vi "HFRR ADV v011 new software.vi"() -> ()   [LabVIEW 2025] (continued)
            n341 = local write "Main Tab"(T2."About" ("Main Tab")) -> ()
            n342 = local write "Cal Password"("" ("Cal Password")) -> ()
            n343 = local write "Main Dashboard Buttons"(T1."About" ("Main Dashboard Buttons")) -> ()
            n344 = local write "Tab Control 5"(T11."Temperature Calibration" ("Tab Control 5")) -> ()
            n345 = property on="Calibration 2" class="TabCtl (strict)"("Visible"=FALSE) -> ()  [unwired: 2 in, 2 out]
            n346 = property on="Tab Control 5" class="TabCtl (strict)"("Tabs Visible?"=FALSE ("Page Labels Display Visible?")) -> ()  [unwired: 2 in, 2 out]
            n347 = local write "Calibration"(FALSE ("Calibration")) -> ()
          }
        }
      }
      event "Calibration Selection": Value Change {
        n348 = event-data() -> ()  [unwired: 1 in, 6 out]
        n349 = local read "Calibration Selection"() -> (w438:T8)
        n350 = case shown="Default" w438 {
          tunnel: [T7."Stroke" ("Main Calibration Tab") T7."Friction" ("Main Calibration Tab") T7."Main" ("Main Calibration Tab") T7."Temperature" ("Main Calibration Tab")] -> w437
          frame "Stroke Calibration" {
          }
          frame "Friction Force Calibration" {
          }
          frame Default {
          }
          frame "Temperature Calibration" {
          }
        }
        n351 = local write "Main Calibration Tab"(w437) -> ()
      }
      event "Back Stroke": Value Change {
        n352 = event-data() -> ()  [unwired: 1 in, 6 out]
        n353 = local write "Main Stroke Tab"(T9."Step 1" ("Main Stroke Tab")) -> ()
        n354 = local write "Main Calibration Tab"(T7."Main" ("Main Calibration Tab")) -> ()
        n355 = local write "Back Stroke"(FALSE ("Back Stroke")) -> ()
      }
      event "Step 2 Back": Value Change {
        n356 = event-data() -> ()  [unwired: 1 in, 6 out]
        n357 = local write "Main Stroke Tab"(T9."Step 1" ("Main Stroke Tab")) -> ()
        n358 = local write "Step 2 Back"(FALSE ("Back Stroke")) -> ()
      }
      event "Step 3 Back": Value Change {
        n359 = event-data() -> ()  [unwired: 1 in, 6 out]
        n360 = local write "Main Stroke Tab"(T9."Step 2" ("Main Stroke Tab")) -> ()
        n361 = local write "Step 3 Back"(FALSE ("Back Stroke")) -> ()
      }
      event "Step 4 Back": Value Change {
        n362 = event-data() -> ()  [unwired: 1 in, 6 out]
        n363 = local write "Main Stroke Tab"(T9."Step 3" ("Main Stroke Tab")) -> ()
        n364 = local write "Step 4 Back"(FALSE ("Back Stroke")) -> ()
      }
      event "Step 5 Back": Value Change {
        n365 = event-data() -> ()  [unwired: 1 in, 6 out]
        n366 = local write "Main Stroke Tab"(T9."Step 4" ("Main Stroke Tab")) -> ()
        n367 = local write "Step 5 Back"(FALSE ("Back Stroke")) -> ()
      }
      event "Step 6 Back": Value Change {
        n368 = event-data() -> ()  [unwired: 1 in, 6 out]
        n369 = local write "Main Stroke Tab"(T9."Step 5" ("Main Stroke Tab")) -> ()
        n370 = local write "Step 6 Back"(FALSE ("Back Stroke")) -> ()
      }
      event "Back Stroke step 7": Value Change {
        n371 = event-data() -> ()  [unwired: 1 in, 6 out]
        n372 = local write "Main Stroke Tab"(T9."Step 6" ("Main Stroke Tab")) -> ()
        n373 = local write "Back Stroke step 7"(FALSE ("Back Stroke")) -> ()
      }
      event "Back Stroke step 8": Value Change {
        n374 = event-data() -> ()  [unwired: 1 in, 6 out]
        n375 = local write "Main Stroke Tab"(T9."Step 7" ("Main Stroke Tab")) -> ()
        n376 = local write "Back Stroke step 8"(FALSE ("Back Stroke")) -> ()
      }
      event "Back Stroke 8": Value Change {
        n377 = event-data() -> ()  [unwired: 1 in, 6 out]
        n378 = local write "Main Stroke Tab"(T9."Step 1" ("Main Stroke Tab")) -> ()
        n379 = local write "Back Stroke 8"(FALSE ("Back Stroke 8")) -> ()
      }
      event "Continue Stroke": Value Change {
        n380 = event-data() -> ()  [unwired: 1 in, 6 out]
        n381 = local write "Main Stroke Tab"(T9."Step 2" ("Main Stroke Tab")) -> ()
        n382 = local write "Continue Stroke"(FALSE ("Continue Stroke")) -> ()
      }
      event "Continue Stroke step 2": Value Change {
        n383 = event-data() -> ()  [unwired: 1 in, 6 out]
        n384 = local write "Main Stroke Tab"(T9."Step 3" ("Main Stroke Tab")) -> ()
        n385 = local write "Continue Stroke step 2"(FALSE ("Continue Stroke")) -> ()
      }
      event "Continue Stroke step 3": Value Change {
        n386 = event-data() -> ()  [unwired: 1 in, 6 out]
        n387 = local write "Main Stroke Tab"(T9."Step 4" ("Main Stroke Tab")) -> ()
        n388 = local write "Continue Stroke step 3"(FALSE ("Continue Stroke")) -> ()
      }
      event "Continue Stroke step 4": Value Change {
        n389 = event-data() -> ()  [unwired: 1 in, 6 out]
        n390 = local write "Main Stroke Tab"(T9."Step 5" ("Main Stroke Tab")) -> ()
        n391 = local write "Continue Stroke step 4"(FALSE ("Continue Stroke")) -> ()
      }
      event "Continue Stroke step 5": Value Change {
        n392 = event-data() -> ()  [unwired: 1 in, 6 out]
        n393 = local write "Main Stroke Tab"(T9."Step 6" ("Main Stroke Tab")) -> ()
        n394 = local write "Continue Stroke step 5"(FALSE ("Continue Stroke")) -> ()
      }
      event "Continue Stroke step 6": Value Change {
        n395 = event-data() -> ()  [unwired: 1 in, 6 out]
        n396 = local write "Main Stroke Tab"(T9."Step 7" ("Main Stroke Tab")) -> ()
        n397 = local write "Continue Stroke step 6"(FALSE ("Continue Stroke")) -> ()
      }
      event "Continue Stroke step 7": Value Change {
        w475 = FALSE ("0.2mm")
        n398 = event-data() -> ()  [unwired: 1 in, 6 out]
        n399 = local write "0.4 mm"(w475) -> ()
        n400 = local write "0.6 mm"(w475) -> ()
        n401 = local write "1.0 mm"(w475) -> ()
        n402 = local write "1.2 mm"(w475) -> ()
        n403 = local write "0.2 2"(w475) -> ()
        n404 = local write "0.4 2"(w475) -> ()
        n405 = local write "0.6 2"(w475) -> ()
        n406 = local write "0.8 2"(w475) -> ()
        n407 = local write "1.0 2"(w475) -> ()
        n408 = local write "1.2"(w475) -> ()
        n409 = local write "0.2mm"(w475) -> ()
        n410 = local write "0.8mm"(w475) -> ()
        n411 = local write "Main Stroke Tab"(T9."Step 8" ("Main Stroke Tab")) -> ()
        n412 = local write "Continue Stroke step 7"(FALSE ("Continue Stroke")) -> ()
        n413 = local write "Stroke Test Complete"(T10."Test Progress" ("Stroke Test Complete")) -> ()
        "Position Measurment Temp" <- 0.0 ("Position Measurment Temp")
        "Calibration Tare" <- TRUE ("Calibration Tare")
      }
      event "Continue Stroke step 8": Value Change {
        n414 = event-data() -> ()  [unwired: 1 in, 6 out]
        n415 = local read "LVDT STROKE  Calibration"() -> (w480:dbl)
        n416 = local read "Position Measurment Temp"() -> (w481:dbl)
        n417 = case shown="0, Default" w481 {
          selector: w481 -> [w486 w491 w496 w501 w506 w511 w514 w517]
          tunnel: w480 -> [w482 w487 w492 w497 w502 w507 _ _]
          frame 0, Default {
            w484 = TRUE ("0.2mm")
            n418 = Increment(x=w486) -> (x+1=w485:i32)
            n419 = local write "Position Measurment Temp"(w485) -> ()
            n420 = local write "0.2mm"(w484) -> ()
            n421 = local write "0.2 2"(w484) -> ()
            n422 = local write "MOVE CARRIAGE TO"(0.2 ("MOVE CARRIAGE TO")) -> ()
            "Calibration 0.2" <- w482
          }
          frame 1 {
            w489 = TRUE ("0.4 mm")
            n423 = Increment(x=w491) -> (x+1=w490:i32)
            n424 = local write "Calibration 0.4"(w487) -> ()
            n425 = local write "Position Measurment Temp"(w490) -> ()
            n426 = local write "0.4 mm"(w489) -> ()
            n427 = local write "MOVE CARRIAGE TO"(0.4 ("MOVE CARRIAGE TO")) -> ()
            n428 = local write "0.4 2"(w489) -> ()
          }
          frame 2 {
            w494 = TRUE ("0.6 mm")
            n429 = Increment(x=w496) -> (x+1=w495:i32)
            n430 = local write "Calibration 0.6"(w492) -> ()
            n431 = local write "Position Measurment Temp"(w495) -> ()
            n432 = local write "0.6 2"(w494) -> ()
            n433 = local write "0.6 mm"(w494) -> ()
            n434 = local write "MOVE CARRIAGE TO"(0.6 ("MOVE CARRIAGE TO")) -> ()
          }
          frame 3 {
            w498 = TRUE ("0.6 mm")
            n435 = Increment(x=w501) -> (x+1=w500:i32)
            n436 = local write "Position Measurment Temp"(w500) -> ()
            n437 = local write "MOVE CARRIAGE TO"(0.8 ("MOVE CARRIAGE TO")) -> ()
            n438 = local write "0.8mm"(w498) -> ()
            n439 = local write "0.8 2"(w498) -> ()
            "Calibration 0.8" <- w497
          }
          frame 4 {
            w503 = TRUE ("0.6 mm")
            n440 = Increment(x=w506) -> (x+1=w505:i32)
            n441 = local write "Position Measurment Temp"(w505) -> ()
            n442 = local write "MOVE CARRIAGE TO"(1.0 ("MOVE CARRIAGE TO")) -> ()
            n443 = local write "1.0 mm"(w503) -> ()
            n444 = local write "1.0 2"(w503) -> ()
            "Calibration 1.0" <- w502
          }
          frame 5 {
            w508 = TRUE ("0.6 mm")
            n445 = Increment(x=w511) -> (x+1=w510:i32)
            n446 = local write "Position Measurment Temp"(w510) -> ()
            n447 = local write "MOVE CARRIAGE TO"(1.2 ("MOVE CARRIAGE TO")) -> ()
            n448 = local write "1.2 mm"(w508) -> ()
            n449 = local write "1.2"(w508) -> ()
            "Calibration 1.2" <- w507
          }
          frame 6 {
            n450 = Increment(x=w514) -> (x+1=w513:i32)
            n451 = local write "Position Measurment Temp"(w513) -> ()
            n452 = local write "Stroke Test Complete"(T10."Stroke Points Completed" ("Stroke Test Complete")) -> ()
          }
          frame 7 {
            n453 = Increment(x=w517) -> (x+1=w516:i32)
            n454 = local write "Position Measurment Temp"(w516) -> ()
            n455 = local write "Main Stroke Tab"(T9."Step 9" ("Main Stroke Tab")) -> ()
          }
        }
      }
      event "Quit": Value Change {
        n456 = event-data() -> ()  [unwired: 1 in, 6 out]
      }
    }
    n457 = Wait (ms)(milliseconds to wait=u32 100) -> ()  [unwired: 1 out]
  }
  n458 = local write "Auto stop temp"(w14) -> ()
  n459 = while {
    stop <- w520 stop-if-true
    n460 = Wait (ms)(milliseconds to wait=u32 200) -> ()  [unwired: 1 out]
    n461 = local read "Quit"() -> (w520:bool)
  }
  n462 = local write "main tab sub"(enum32{"Page 1", "Page 2"}."Page 1" ("main tab sub")) -> ()
  n463 = local write "USERNAME"(w31) -> ()
  n464 = local write "Main Tab"(T2."HOME" ("Main Tab")) -> ()
  n465 = local write "USER ID"(w31) -> ()
  n466 = property on="Auto Scar Check  2" class="Clust (strict)"("Visible"=w14) -> (error out=w17:errorcluster)  [unwired: 2 in, 1 out]
  n467 = property on="Quit" class="Bool (strict)"("Value"=FALSE ("Quit")) -> (error out=w33:errorcluster)  [unwired: 2 in, 1 out]
  n468 = while {
    shift-right: [w522] -> _
    shift-left: "Enum - Selector" -> [w523]
    stop <- w524 stop-if-true
    # "Auto Start Logic Loop"
    n469 = case shown="\"close\"" w523 {
      tunnel: [w527 w533 w560 w592 w622 Auto_Start_enum."Exit" ("Enum - Selector") Auto_Start_enum."Init" ("Enum - Selector")] -> w522
      frame "Init", Default {
        n470 = local read "Auto Start Test"() -> (w526:bool)
        n471 = Select(t=Auto_Start_enum."Humidity & Temperature On" ("Enum - Selector"), s=w526, f=Auto_Start_enum."Init") -> (s? t:f=w527:T14)
      }
      frame "Humidity & Temperature On" {
        n472 = stacked-sequence {
          tunnel: [_ _ _ _ _ _ Auto_Start_enum."Reach point" ("Enum - Selector")] -> w530
          frame #0 {
            w535 = T17."Disabled and Grayed Out" ("Disabled")
            w536 = TRUE ("Heater Button")
            n473 = property on="Humidity" class="Bool (strict)"("DisabledEnum"=w535) -> ()  [unwired: 2 in, 2 out]
            n474 = property on="Heater Button" class="Bool (strict)"("DisabledEnum"=w535) -> ()  [unwired: 2 in, 2 out]
            n475 = local write "Heater Button"(w536) -> ()
            n476 = local write "Humidity"(w536) -> ()
            n477 = property on="Heater Button" class="Bool (strict)"("Val(Sgnl)"=TRUE ("Value (Signaling)")) -> ()  [unwired: 2 in, 2 out]
          }
          frame #1 {
            n478 = Wait (ms)(milliseconds to wait=u32 3000) -> ()  [unwired: 1 out]
          }
          frame #2 {
            n479 = local read "Set Temp"() -> (w542:dbl)
            n480 = Number To Fractional String(number=w542, precision (6)=i16 2) -> (F-format string=w539:string)  [unwired: 2 in]
            n481 = Concatenate Strings("ST;" ("Command"), w539) -> (w540:string)
            n482 = local write "Command"(w540) -> ()
          }
          frame #3 {
            n483 = Wait (ms)(milliseconds to wait=u32 1500) -> ()  [unwired: 1 out]
          }
          frame #4 {
            (unwired) i16 2 ("precision (6)")
            n484 = local read "Set Rh"() -> (w545:dbl)
            n485 = Number To Fractional String(number=w545) -> (F-format string=w548:string)  [unwired: 3 in]
            n486 = local read "WriteHumidity"() -> (w546:string[])
            n487 = Concatenate Strings("M;" ("new element/subarray"), w548) -> (w549:string)
            n488 = local write "Command"("HE;1" ("Command")) -> ()
            n489 = Insert Into Array(array=w546, new element=w549) -> (w547:string[])  [unwired: 1 in]
            n490 = local write "WriteHumidity"(w547) -> ()
          }
          frame #5 {
            n491 = Wait (ms)(milliseconds to wait=u32 1500) -> ()  [unwired: 1 out]
          }
          frame #6 {
            w552 = TRUE ("Reach point temp")
            n492 = local write "Reach point Humidity"(w552) -> ()
            n493 = local write "Reach point temp"(w552) -> ()
          }
        }
        n494 = local read "Auto Start Test"() -> (w532:bool)
        n495 = Not(x=w532) -> (.not. x?=w531:bool)
        n496 = Select(t=Auto_Start_enum."close", s=w531, f=w530) -> (s? t:f=w533:T14)
      }
      frame "Reach point" {
        w561 = TRUE ("PAUSE")
        w569 = 1.0 ("y")
        w572 = 1.0 ("y")
        n497 = local read "Set Temp"() -> (w554:dbl)
        n498 = local read "Set Humidity:"() -> (w568:dbl)
        n499 = local read "Humidity ( %RH )"() -> (w573:dbl)
        n500 = Add(x=w554, y=w572) -> (x+y=w571:dbl)
        n501 = Subtract(x=w554, y=w572) -> (x-y=w570:dbl)
        n502 = Add(x=w568, y=w569) -> (x+y=w567:dbl)
        n503 = Subtract(x=w568, y=w569) -> (x-y=w566:dbl)
        n504 = local read "TEMP"() -> (w574:dbl)
        n505 = In Range and Coerce(upper limit=w567, x=w573, lower limit=w566) -> (In Range?=w555:bool)  [unwired: 1 out]
        n506 = In Range and Coerce(upper limit=w571, x=w574, lower limit=w570) -> (In Range?=w556:bool)  [unwired: 1 out]
        n507 = case shown="True" w555 {
          frame False {
          }
          frame True {
            n508 = case shown="True" "Reach point Humidity" {
              selector: "Reach point Humidity" -> [_ w580]
              frame False {
              }
              frame True {
                n509 = local read "EVENT LOG"() -> (w577:string)
                n510 = Not(x=w580) -> (.not. x?=w579:bool)
                n511 = local write "Reach point Humidity"(w579) -> ()
                n512 = call "Event Log.vi"("Content"="Target Humidity reached", "EVENT LOG"=w577) -> ("EVENT LOG"=w578:string)  [unwired: 8 in, 1 out]
                n513 = local write "EVENT LOG"(w578) -> ()
              }
            }
          }
        }
        n514 = case shown="True" w556 {
          frame False {
          }
          frame True {
            n515 = case shown="True" "Reach point temp" {
              selector: "Reach point temp" -> [_ w586]
              frame False {
              }
              frame True {
                n516 = local read "EVENT LOG"() -> (w583:string)
                n517 = Not(x=w586) -> (.not. x?=w585:bool)
                n518 = local write "Reach point temp"(w585) -> ()
                n519 = call "Event Log.vi"("Content"="Target Temperature reached", "EVENT LOG"=w583) -> ("EVENT LOG"=w584:string)  [unwired: 8 in, 1 out]
                n520 = local write "EVENT LOG"(w584) -> ()
              }
            }
          }
        }
        n521 = local read "Auto Start Test"() -> (w559:bool)
        n522 = And(x=w556, y=w555) -> (x .and. y?=w565:bool)
        n523 = Select(t=Auto_Start_enum."Maintain Stage" ("Enum - Selector"), s=w565, f=Auto_Start_enum."Reach point" ("Enum - Selector")) -> (s? t:f=w562:T14)
        n524 = Not(x=w559) -> (.not. x?=w558:bool)
        n525 = Select(t=Auto_Start_enum."close", s=w558, f=w562) -> (s? t:f=w560:T14)
        n526 = call "ELAPSED TIMER VI.vi"("RESET"=w561, "PAUSE"=w561) -> ()  [unwired: 7 in, 3 out]
      }
      frame "Maintain Stage" {
        w601 = 2.0 ("y")
        w600 = 1.0 ("y")
        # "Humidity and  temperatures Set Point  have been reached"
        n527 = local read "Set Temp"() -> (w587:dbl)
        n528 = local read "Set Humidity:"() -> (w604:dbl)
        n529 = local read "Humidity ( %RH )"() -> (w607:dbl)
        n530 = Add(x=w587, y=w600) -> (x+y=w606:dbl)
        n531 = Subtract(x=w587, y=w600) -> (x-y=w605:dbl)
        n532 = local read "TEMP"() -> (w608:dbl)
        n533 = Add(x=w604, y=w601) -> (x+y=w603:dbl)
        n534 = Subtract(x=w604, y=w601) -> (x-y=w602:dbl)
        n535 = In Range and Coerce(upper limit=w606, x=w608, lower limit=w605) -> (In Range?=w599:bool)  [unwired: 1 out]
        n536 = In Range and Coerce(upper limit=w603, x=w607, lower limit=w602) -> (In Range?=w598:bool)  [unwired: 1 out]
        n537 = And(x=w599, y=w598) -> (x .and. y?=w597:bool)
        n538 = Not(x=w597) -> (.not. x?=w596:bool)
        n539 = call "ELAPSED TIMER VI.vi"("TARGET"=60.0, "RESET"=w596, "PAUSE"=FALSE) -> ("ELAPSED INDICATION"=w593:bool)  [unwired: 6 in, 2 out]
        n540 = case shown="True" w593 {
          tunnel: w593 -> [_ w611]
          tunnel: [Auto_Start_enum."Maintain Stage" ("Enum - Selector") w610] -> w591
          frame False {
          }
          frame True {
            n541 = stacked-sequence {
              tunnel: w611 -> [_ _ _ _ _]
              tunnel: [_ _ _ _ Auto_Start_enum."Start Stage" ("Enum - Selector")] -> w610
              frame #0 {
                n542 = local read "EVENT LOG"() -> (w613:string)
                n543 = call "Event Log.vi"("Content"="Humidity and temperature set point has stabilized.", "EVENT LOG"=w613) -> ("EVENT LOG"=w614:string)  [unwired: 8 in, 1 out]
                n544 = local write "EVENT LOG"(w614) -> ()
              }
              frame #1 {
                n545 = Wait (ms)(milliseconds to wait=u32 100) -> ()  [unwired: 1 out]
              }
              frame #2 {
                n546 = local read "EVENT LOG"() -> (w617:string)
                n547 = call "Event Log.vi"("Content"="Auto Test Started", "EVENT LOG"=w617) -> ("EVENT LOG"=w618:string)  [unwired: 8 in, 1 out]
                n548 = local write "EVENT LOG"(w618) -> ()
              }
              frame #3 {
                w619 = TRUE ("RUN")
                n549 = local write "RUN"(w619) -> ()
                n550 = property on="Auto Start Temp" class="Bool (strict)"("Val(Sgnl)"=w619) -> ()  [unwired: 2 in, 2 out]
                "Auto Start Temp" <- w619
              }
              frame #4 {
              }
            }
          }
        }
        n551 = local read "Auto Start Test"() -> (w590:bool)
        n552 = Not(x=w590) -> (.not. x?=w589:bool)
        n553 = Select(t=Auto_Start_enum."close", s=w589, f=w591) -> (s? t:f=w592:T14)
      }
      frame "Start Stage" {
        w621 = TRUE ("PAUSE")
        n554 = local read "Auto Start Test"() -> (w626:bool)
        n555 = Not(x=w626) -> (.not. x?=w625:bool)
        n556 = Select(t=Auto_Start_enum."close" ("Enum - Selector"), s=w625, f=Auto_Start_enum."Start Stage" ("Enum - Selector")) -> (s? t:f=w622:T14)
        n557 = call "ELAPSED TIMER VI.vi"("RESET"=w621, "PAUSE"=w621) -> ()  [unwired: 7 in, 3 out]
      }
      frame "close" {
        w628 = FALSE ("Heater Button")
        n558 = local write "RUN"(w628) -> ()
        n559 = local write "Heater Button"(w628) -> ()
        n560 = local write "Humidity"(w628) -> ()
        n561 = local write "Auto Start Test"(w628) -> ()
        n562 = property on="Heater Button" class="Bool (strict)"("Val(Sgnl)"=FALSE ("Value (Signaling)")) -> ()  [unwired: 2 in, 2 out]
      }
      frame "Exit" {
      }
    }
    n563 = Wait (ms)(milliseconds to wait=u32 100) -> ()  [unwired: 1 out]
    n564 = local read "Quit"() -> (w524:bool)
  }
  n565 = property on="Service Password Log" class="Str"("Visible"=w14) -> ()  [unwired: 2 in, 2 out]
  n566 = property on="Password 3" class="Clust (strict)"("Visible"=w14) -> ()  [unwired: 2 in, 2 out]
  n567 = while {
    stop <- w657 stop-if-true
    w640 = errorcluster {"status"=FALSE, "code"=0, "source"=""} ("error in (no error) 3")
    # "this loop is for manual report generation"
    n568 = local read "Confirm Measrurement"() -> (w639:bool)
    n569 = case shown="True" w639 {
      selector: w639 -> [_ w747]
      tunnel: errorcluster {"status"=FALSE, "code"=0, "source"=""} ("error in (no error) 3") -> [_ w748]
      tunnel: [_ w746] -> _
      frame False {
      }
      frame True {
        n570 = stacked-sequence {
          tunnel: w748 -> [_ w781 _]
          tunnel: w747 -> [_ _ w888]
          tunnel: [_ w769 _] -> w746
          frame #0 {
            n571 = String To Path(string="C:\\LAB-IQ\\Image Calibrate v01.dcf") -> (path=w751:path)
            n572 = Open/Create/Replace File ("Open File")(file path (use dialog)=w751) -> (refnum out=w752:refnum<file>)  [unwired: 5 in, 2 out]
            n573 = for {
              N: 4 -> [_]
              tunnel: w752 -> [w758]
              i -> [w754]
              n574 = Read from Text File ("Read File")(file (use dialog)=w758) -> (text=w759:string)  [unwired: 3 in, 3 out]
              n575 = String Subset(string=w759, offset (0)=6, length (rest)=10 ("length (rest)")) -> (substring=w755:string)
              n576 = Fract/Exp String To Number(string=w755) -> (number=w753:dbl)  [unwired: 3 in, 1 out]
              n577 = case shown="3" w754 {
                tunnel: w753 -> [w760 w761 _ w762 _]
                frame 0 {
                  n578 = local write "5x Gain"(w760) -> ()
                }
                frame 1 {
                  n579 = local write "10x Gain"(w761) -> ()
                }
                frame 2 {
                }
                frame 3 {
                  n580 = local write "100x gain"(w762) -> ()
                }
                frame 4, Default {
                }
              }
            }
          }
          frame #1 {
            n581 = local read "TEST STANDARD"() -> (w764:T3)
            n582 = case shown="\"ISO 12156\"" w764 {
              tunnel: ["ASTM D6079" "ISO 12156"] -> w763
              frame "ASTM D6079", Default {
              }
              frame "ISO 12156" {
              }
            }
            n583 = call "IMAGE ANALYSIS.vi"("Enum"=POST_ANALYSIS_ENUM."GET MEASUREMENTS", "error in"=w781) -> ("error out"=w788:errorcluster)  [unwired: 8 in, 1 out]
            n584 = local read "Magnification :"() -> (w774:string)
            n585 = call "Stall Data Flow.vim"("value in"=w788, "milliseconds to wait"=u32 1000) -> ("value out"=w787:errorcluster)  [unwired: 1 out]
            n586 = local read "Test File List :"() -> (w785:string)
            n587 = case shown="\"10x\"" w774 {
              tunnel: [w824 w825] -> w772
              frame "5x", Default {
                n588 = local read "5x Gain"() -> (w824:dbl)
              }
              frame "10x" {
                # "5x"
                n589 = local read "10x Gain"() -> (w825:dbl)
              }
            }
            n590 = call "IMAGE ANALYSIS.vi"("Enum"=POST_ANALYSIS_ENUM."READ", "error in"=w787) -> ("error out"=w784:errorcluster, "data out"=w775:string)  [unwired: 8 in]
            n591 = Match Pattern(string=w775, regular expression="\"type\": ") -> (after substring=w779:string)  [unwired: 1 in, 3 out]
            n592 = call "IMAGE PATH CREATION PY.vi"("error in (no error)"=w784, "File Name :"=w785) -> ("error out"=w783:errorcluster, "File Path"=w771:path, "File Path String:"=w766:string)  [unwired: 7 in]
            n593 = Match Pattern(string=w779, regular expression=",") -> (before substring=w765:string)  [unwired: 1 in, 3 out]
            n594 = local read "Calibration Tab"() -> (w768:enum32{"Measrument", "Calibrate"})
            n595 = call "Stall Data Flow.vim"("value in"=w783, "milliseconds to wait"=u32 250) -> ("value out"=w767:errorcluster)  [unwired: 1 out]
            n596 = Equal?(x=w765, y="\"rectangle\"") -> (x = y?=w776:bool)
            n597 = case shown="False" w776 {
              tunnel: w775 -> [w830 w885]
              tunnel: w772 -> [_ w876]
              tunnel: cluster{"major":dbl, "minor":dbl, "average":dbl} {"major"=0.0, "minor"=0.0, "average"=0.0} -> [w828 w872]
              tunnel: [w827 w869] -> w770
              tunnel: w765 -> [w829 _]
              tunnel: w772 -> [w826 _]
              frame False {
                n598 = Equal?(x=w829, y="\"line\"") -> (x = y?=w831:bool)
                n599 = case shown="True" w831 {
                  tunnel: w830 -> [_ w846]
                  tunnel: w828 -> [w833 w845]
                  tunnel: [w833 w843] -> w827
                  tunnel: w826 -> [_ w842]
                  frame False {
                  }
                  frame True {
                    w841 = 0.0 ("Major Axis")
                    n600 = Match Pattern(string=w846, regular expression="\"length_px\":") -> (after substring=w844:string)  [unwired: 1 in, 3 out]
                    n601 = property on="Major Axis" class="DigNum (strict)"("Caption.Text"="") -> ()  [unwired: 2 in, 2 out]
                    n602 = property on="Minor Axis" class="DigNum (strict)"("Caption.Text"="") -> ()  [unwired: 2 in, 2 out]
                    n603 = property on="Average" class="DigNum (strict)"("Caption.Text"="Line") -> ()  [unwired: 2 in, 2 out]
                    n604 = Fract/Exp String To Number(string=w844, default (0 dbl)=0.0 ("default (0 DBL)")) -> (number=w840:dbl)  [unwired: 2 in, 1 out]
                    "Pixel Value" <- w840
                    n605 = Multiply(x=w840, y=w842) -> (x*y=w853:dbl)
                    n606 = Multiply(x=w853, y=1000.0) -> (x*y=w836:dbl)
                    n607 = Divide(x=w836, y=1000.0) -> (x/y=w839:dbl)
                    n608 = local write "Measurment (mm)"(w839) -> ()
                    n609 = Bundle By Name(cluster=w845, "average"=w836) -> (w843:cluster{"major":dbl, "minor":dbl, "average":dbl})
                    n610 = Number To Fractional String(number=w836, precision (6)=i16 1) -> (F-format string=w835:string)  [unwired: 2 in]
                    n611 = local write "Minor Axis"(w841) -> ()
                    n612 = local write "Major Axis"(w841) -> ()
                    n613 = Fract/Exp String To Number(string=w835) -> (number=w834:dbl)  [unwired: 3 in, 1 out]
                    n614 = local write "Average"(w834) -> ()
                  }
                }
              }
              frame True {
                w873 = 1000.0 ("y")
                w879 = 0.0 ("default (0 DBL)")
                n615 = Match Pattern(string=w885, regular expression=" \"width_px\":") -> (after substring=w883:string)  [unwired: 1 in, 3 out]
                n616 = Match Pattern(string=w883, regular expression="\"height_px\":") -> (before substring=w881:string, after substring=w880:string)  [unwired: 1 in, 2 out]
                n617 = Fract/Exp String To Number(string=w881, default (0 dbl)=w879) -> (number=w878:dbl)  [unwired: 2 in, 1 out]
                n618 = Fract/Exp String To Number(string=w880, default (0 dbl)=w879) -> (number=w877:dbl)  [unwired: 2 in, 1 out]
                n619 = Multiply(x=w878, y=w876) -> (x*y=w875:dbl)
                n620 = Multiply(x=w877, y=w876) -> (x*y=w874:dbl)
                n621 = Multiply(x=w875, y=w873) -> (x*y=w859:dbl)
                n622 = Multiply(x=w874, y=w873) -> (x*y=w857:dbl)
                n623 = Add(x=w859, y=w857) -> (x+y=w871:dbl)
                n624 = property on="Major Axis" class="DigNum (strict)"("Caption.Text"="Major Axis") -> ()  [unwired: 2 in, 2 out]
                n625 = property on="Minor Axis" class="DigNum (strict)"("Caption.Text"="Minor Axis") -> ()  [unwired: 2 in, 2 out]
                n626 = property on="Average" class="DigNum (strict)"("Caption.Text"="Average") -> ()  [unwired: 2 in, 2 out]
                n627 = Divide(x=w871, y=2.0) -> (x/y=w855:dbl)
                n628 = Bundle By Name(cluster=w872, "major"=w859, "minor"=w857, "average"=w855) -> (w869:cluster{"major":dbl, "minor":dbl, "average":dbl})
                n629 = Number To Fractional String(number=w857, precision (6)=i16 1) -> (F-format string=w864:string)  [unwired: 2 in]
                n630 = Number To Fractional String(number=w855, precision (6)=i16 1) -> (F-format string=w865:string)  [unwired: 2 in]
                n631 = Number To Fractional String(number=w859, precision (6)=i16 1) -> (F-format string=w863:string)  [unwired: 2 in]
                n632 = Fract/Exp String To Number(string=w864) -> (number=w856:dbl)  [unwired: 3 in, 1 out]
                n633 = Fract/Exp String To Number(string=w865) -> (number=w854:dbl)  [unwired: 3 in, 1 out]
                n634 = Fract/Exp String To Number(string=w863) -> (number=w858:dbl)  [unwired: 3 in, 1 out]
                n635 = local write "Major Axis"(w858) -> ()
                n636 = local write "Average"(w854) -> ()
                n637 = local write "Minor Axis"(w856) -> ()
              }
            }
            n638 = case shown="\"Measrument\", Default" w768 {
              tunnel: w771 -> [w798 _]
              tunnel: w770 -> [w797 _]
              tunnel: [w794 w823] -> w769
              tunnel: w767 -> [w796 w823]
              tunnel: w766 -> [w795 _]
              tunnel: w763 -> [w793 _]
              frame "Measrument", Default {
                n639 = stacked-sequence {
                  tunnel: w798 -> [w816 _]
                  tunnel: w797 -> [w814 _]
                  tunnel: w796 -> [w812 _]
                  tunnel: w795 -> [w811 _]
                  tunnel: [w806 _] -> w794
                  tunnel: w793 -> [w799 _]
                  frame #0 {
                    n640 = call "IMAGE ANALYSIS.vi"("Enum"=POST_ANALYSIS_ENUM."SAVE IMAGE", "error in"=w812, "IMAGE FILE PATH"=w811) -> ("error out"=w810:errorcluster)  [unwired: 7 in, 1 out]
                    n641 = call "Stall Data Flow.vim"("value in"=w810, "milliseconds to wait"=u32 1000) -> ("value out"=w801:errorcluster)  [unwired: 1 out]
                    n642 = local read "Test File List :"() -> (w818:string)
                    n643 = call "IMAGE ANALYSIS.vi"("Enum"=POST_ANALYSIS_ENUM."MINIMIZE UI", "error in"=w801) -> ("error out"=w808:errorcluster)  [unwired: 8 in, 1 out]
                    n644 = Bundle By Name(cluster=T24 {"File Name"="", "Test Method"="", "Operator"="", "Fuel Description"="", "Date and time"=""} ("Main Ref"), "Test Method"=w799, "File Name"=w818) -> (w819:T24)
                    n645 = call "Stall Data Flow.vim"("value in"=w808, "milliseconds to wait"=u32 1500) -> ("value out"=w803:errorcluster)  [unwired: 1 out]
                    n646 = call "duf file read.vi"("error in (no error)"=w803, "Main Ref"=w819) -> ("error out"=w817:errorcluster, "Main Ref 2"=w815:T24)  [unwired: 8 in]
                    n647 = call "DETECTION REPORT for manual.vi"("error in (no error)"=w817, "return value 3"=w814, "Image File Path"=w816, "Main Ref"=w815) -> ("error out"=w813:errorcluster)  [unwired: 7 in]
                    n648 = call <vilib>:"Clear Errors.vi"("error in (no error)"=w813) -> ("error out"=w804:errorcluster)  [unwired: 5 in, 1 out]
                    n649 = call "IMAGE ANALYSIS.vi"("Enum"=POST_ANALYSIS_ENUM."MINIMIZE UI", "error in"=w804) -> ("error out"=w806:errorcluster)  [unwired: 8 in, 1 out]
                  }
                  frame #1 {
                    n650 = local write "Main Tab"(T2."HOME" ("Main Tab")) -> ()
                    n651 = local write "Main Dashboard Buttons"(T1."Home" ("Main Dashboard Buttons")) -> ()
                  }
                }
              }
              frame "Calibrate" {
              }
            }
          }
          frame #2 {
            n652 = Not(x=w888) -> (.not. x?=w887:bool)
            n653 = local write "Confirm Measrurement"(w887) -> ()
            n654 = local read "Calibration Tab"() -> (w886:enum32{"Measrument", "Calibrate"})
            n655 = case shown="\"Measrument\", Default" w886 {
              frame "Measrument", Default {
                (unwired) T19."HOME" ("Main Tab")
                n656 = local write "Main Tab"(T2."HOME" ("Main Tab")) -> ()
              }
              frame "Calibrate" {
              }
            }
          }
        }
      }
    }
    n657 = local read "Humidity"() -> (w631:bool)
    n658 = local read "Save Change"() -> (w636:bool)
    n659 = local read "Calibrate"() -> (w637:bool)
    n660 = local read "Auto Start Test"() -> (w632:bool)
    n661 = case shown="True" w637 {
      selector: w637 -> [_ w744]
      frame False {
      }
      frame True {
        n662 = Not(x=w744) -> (.not. x?=w743:bool)
        n663 = local write "Calibrate"(w743) -> ()
        n664 = local write "Calibration Tab"(enum32{"Measrument", "Calibrate"}."Calibrate" ("Calibration Tab")) -> ()
      }
    }
    n665 = case shown="True" w636 {
      selector: w636 -> [_ w688]
      frame False {
      }
      frame True {
        n666 = stacked-sequence {
          tunnel: w688 -> [_ _ _ _ w742]
          frame #0 {
            n667 = call "IMAGE ANALYSIS.vi"("Enum"=POST_ANALYSIS_ENUM."HIDE UI") -> ()  [unwired: 9 in, 2 out]
          }
          frame #1 {
            n668 = local read "100x gain"() -> (w690:dbl)
            n669 = local read "10x Gain"() -> (w691:dbl)
            n670 = local read "5x Gain"() -> (w692:dbl)
            n671 = Number To Fractional String(number=w691, width (-)=i16 4, precision (6)=i16 7) -> (F-format string=w713:string)  [unwired: 1 in]
            n672 = Number To Fractional String(number=0.0, width (-)=i16 4, precision (6)=i16 7) -> (F-format string=w708:string)  [unwired: 1 in]
            n673 = Number To Fractional String(number=w690, width (-)=i16 4, precision (6)=i16 7) -> (F-format string=w696:string)  [unwired: 1 in]
            n674 = Number To Fractional String(number=w692, width (-)=i16 10 ("precision (6)"), precision (6)=i16 7) -> (F-format string=w722:string)  [unwired: 1 in]
            n675 = Concatenate Strings("[CH1]" ("string"), w722, " - 5x Gain" ("string"), "\r") -> (w712:string)
            n676 = Concatenate Strings("[CH2]" ("string"), w713, " - 10x Gain" ("string"), "\r") -> (w711:string)
            n677 = Concatenate Strings("[CH3]" ("string"), w708, " - 20x Gain" ("string"), "\r") -> (w702:string)
            n678 = Concatenate Strings("[CH4]" ("string"), w696, " - 100x Gain" ("string"), "\r") -> (w695:string)
            n679 = String To Path(string="C:\\LAB-IQ\\Image Calibrate v01.dcf") -> (path=w725:path)
            n680 = Concatenate Strings(w712, w711, w702, w695) -> (w710:string)
            n681 = call <vilib>:"Write Characters To File.vi"("append to file? (new file:F)"=FALSE, "character string"=w710, "file path (dialog if empty)"=w725) -> ()  [unwired: 2 in, 1 out]
          }
          frame #2 {
            n682 = String To Path(string="C:\\LAB-IQ\\Image Calibrate v01.dcf") -> (path=w728:path)
            n683 = Open/Create/Replace File ("Open File")(file path (use dialog)=w728) -> (refnum out=w729:refnum<file>)  [unwired: 5 in, 2 out]
            n684 = for {
              N: 4 -> [_]
              tunnel: w729 -> [w735]
              i -> [w731]
              n685 = Read from Text File ("Read File")(file (use dialog)=w735) -> (text=w736:string)  [unwired: 3 in, 3 out]
              n686 = String Subset(string=w736, offset (0)=6, length (rest)=10 ("length (rest)")) -> (substring=w732:string)
              n687 = Fract/Exp String To Number(string=w732) -> (number=w730:dbl)  [unwired: 3 in, 1 out]
              n688 = case shown="3" w731 {
                tunnel: w730 -> [w737 w738 _ w739 _]
                frame 0 {
                  n689 = local write "5x Gain"(w737) -> ()
                }
                frame 1 {
                  n690 = local write "10x Gain"(w738) -> ()
                }
                frame 2 {
                }
                frame 3 {
                  n691 = local write "100x gain"(w739) -> ()
                }
                frame 4, Default {
                }
              }
            }
          }
          frame #3 {
            n692 = call "IMAGE ANALYSIS.vi"("Enum"=POST_ANALYSIS_ENUM."SHOW UI") -> ()  [unwired: 9 in, 2 out]
          }
          frame #4 {
            n693 = Not(x=w742) -> (.not. x?=w741:bool)
            n694 = local write "Save Change"(w741) -> ()
          }
        }
      }
    }
    n695 = case shown="False" w632 {
      tunnel: w631 -> [w658 _]
      frame False {
        n696 = case shown="True" w658 {
          frame False {
          }
          frame True {
            n697 = local read "Set Humidity:"() -> (w662:dbl)
            n698 = local read "Set Humidity:"() -> (w665:dbl)
            n699 = local read "Humidity ( %RH )"() -> (w666:dbl)
            n700 = Subtract(x=w662, y=2.0) -> (x-y=w660:dbl)
            n701 = Add(x=w665, y=2.0) -> (x+y=w661:dbl)
            n702 = In Range and Coerce(upper limit=w661, x=w666, lower limit=w660) -> (In Range?=w659:bool)  [unwired: 1 out]
            n703 = case shown="True" w659 {
              frame False {
              }
              frame True {
                n704 = case shown="True" "Manual Humididty Reached" {
                  selector: "Manual Humididty Reached" -> [_ w669]
                  frame False {
                  }
                  frame True {
                    n705 = Not(x=w669) -> (.not. x?=w668:bool)
                    n706 = local write "Manual Humididty Reached"(w668) -> ()
                    n707 = local read "EVENT LOG"() -> (w671:string)
                    n708 = call "Event Log.vi"("Content"="Target Humidity reached", "EVENT LOG"=w671) -> ("EVENT LOG"=w670:string)  [unwired: 8 in, 1 out]
                    n709 = local write "EVENT LOG"(w670) -> ()
                  }
                }
              }
            }
          }
        }
      }
      frame True {
        n710 = local write "Manual Humididty Reached"(TRUE ("Manual Humididty Reached")) -> ()
      }
    }
    n711 = local read "Cap Live Image"() -> (w652:bool)
    n712 = local read "SCAR MEASURMENT"() -> (w655:enum32{"Auto Scar", "Manual Scar"})
    n713 = Wait (ms)(milliseconds to wait=u32 250) -> ()  [unwired: 1 out]
    n714 = Equal?(x=w655, y=enum32{"Auto Scar", "Manual Scar"}."Manual Scar" ("SCAR MEASURMENT")) -> (x = y?=w653:bool)
    n715 = And(x=w653, y=w652) -> (x .and. y?=w651:bool)
    n716 = case shown="True" w651 {
      selector: w651 -> [_ w967]
      frame False {
      }
      frame True {
        n717 = stacked-sequence {
          tunnel: [_ _ _ w982 _] -> _
          tunnel: w967 -> [_ _ _ _ w989]
          frame #0 {
            w968 = 0.0
            n718 = local write "Major Axis"(w968) -> ()
            n719 = local write "Minor Axis"(w968) -> ()
            n720 = local write "Average"(w968) -> ()
          }
          frame #1 {
            n721 = call "CAMERA LIVE FEED FGV.vi"("Enum - Menu"=CAMERA_LIVE_FEED_ENUM."CAMERA MINIMIZE") -> ()  [unwired: 9 in, 2 out]
          }
          frame #2 {
            n722 = local read "FILE 3"() -> (w976:string)
            n723 = call <vilib>:"Trim Whitespace.vi"("string"="C:\\LAB-IQ\\images\\") -> ("trimmed string"=w978:string)  [unwired: 1 in]
            n724 = String To Path(string=w978) -> (path=w977:path)
            n725 = Concatenate Strings(w976, ".png" ("string")) -> (w975:string)
            n726 = Build Path(base path=w977, name or relative path=w975) -> (appended path=w973:path)
            n727 = Path To String(path=w973) -> (string=w972:string)
            n728 = call "CAMERA LIVE FEED FGV.vi"("Enum - Menu"=CAMERA_LIVE_FEED_ENUM."CAMERA SAVE", "Image Path"=w972) -> ("error out"=w970:errorcluster)  [unwired: 8 in, 1 out]
            n729 = case shown="No Error" w970 {
              frame No Error {
                n730 = One Button Dialog(message="Image saved successfully") -> ()  [unwired: 1 in, 1 out]
              }
              frame Error {
              }
            }
          }
          frame #3 {
            n731 = call "LIST FILE NAMES.vi"() -> ("error out"=w984:errorcluster, "filenames"=w981:string[])  [unwired: 10 in]
            n732 = call "IMAGE ANALYSIS.vi"("Enum"=POST_ANALYSIS_ENUM."SHOW UI", "error in"=w984) -> ("error out"=w982:errorcluster)  [unwired: 8 in, 1 out]
            n733 = property on="Test File List :" class="CmbBox"("Strings[]"=w981) -> ()  [unwired: 2 in, 2 out]
          }
          frame #4 {
            (unwired) T23."Report" ("Main Dashboard Buttons")
            (unwired) T25."Report" ("Main Dashboard Buttons")
            n734 = Not(x=w989) -> (.not. x?=w988:bool)
            n735 = local write "Zoom Factore"(0.0 ("Zoom Factore")) -> ()
            n736 = local write "Cap Live Image"(w988) -> ()
            n737 = local write "Main Tab"(T2."Adv Scar Report" ("Main Tab")) -> ()
            n738 = property on="Cap Live Image" class="Bool (strict)"("BoolText.Text"="Capture Image" ("Boolean Text.Text")) -> ()  [unwired: 2 in, 2 out]
            n739 = local write "Main Dashboard Buttons"(T1."Report" ("Main Dashboard Buttons")) -> ()
          }
        }
      }
    }
    n740 = local read "change Gain"() -> (w635:bool)
    n741 = local read "Back Square"() -> (w634:bool)
    n742 = case shown="True" w635 {
      selector: w635 -> [_ w679]
      frame False {
      }
      frame True {
        n743 = stacked-sequence {
          tunnel: w679 -> [_ w687]
          frame #0 {
            n744 = local read "Actual (µm)"() -> (w683:dbl)
            n745 = local read "Pixel Value"() -> (w682:dbl)
            n746 = local read "Magnification :"() -> (w681:string)
            n747 = Divide(x=w683, y=w682) -> (x/y=w680:dbl)
            n748 = case shown="\"10x\"" w681 {
              tunnel: w680 -> [w684 w685]
              frame "10x" {
                n749 = local write "10x Gain"(w684) -> ()
              }
              frame "5x", Default {
                n750 = local write "5x Gain"(w685) -> ()
              }
            }
          }
          frame #1 {
            n751 = Not(x=w687) -> (.not. x?=w686:bool)
            n752 = local write "change Gain"(w686) -> ()
          }
        }
      }
    }
    n753 = case shown="True" w634 {
      selector: w634 -> [_ w677]
      frame False {
      }
      frame True {
        n754 = Not(x=w677) -> (.not. x?=w676:bool)
        n755 = local write "Back Square"(w676) -> ()
        n756 = local write "Calibration Tab"(enum32{"Measrument", "Calibrate"}."Measrument" ("Calibration Tab")) -> ()
      }
    }
    n757 = local read "Rectangle Tool"() -> (w646:bool)
    n758 = local read "Clear ROI Tool"() -> (w645:bool)
    n759 = local read "Open Image"() -> (w650:bool)
    n760 = local read "line tool"() -> (w647:bool)
    n761 = local read "OUT"() -> (w648:bool)
    n762 = local read "In"() -> (w649:bool)
    n763 = case shown="True" w650 {
      selector: w650 -> [_ w955]
      tunnel: [w951 w957] -> _
      tunnel: w640 -> [w951 w956]
      frame False {
      }
      frame True {
        n764 = Not(x=w955) -> (.not. x?=w954:bool)
        n765 = local write "Open Image"(w954) -> ()
        n766 = call "IMAGE ANALYSIS.vi"("Enum"=POST_ANALYSIS_ENUM."HIDE UI", "error in"=w956) -> ("error out"=w964:errorcluster)  [unwired: 8 in, 1 out]
        n767 = call "File Dialog"("start path"=path "C:/LAB-IQ/images", "error in"=w964) -> ("selected path"=w953:path, "error out"=w962:errorcluster)  [unwired: 10 in, 2 out]
        "Image path  2" <- w953
        n768 = call <vilib>:"Clear Errors.vi"("error in (no error)"=w962) -> ("error out"=w961:errorcluster)  [unwired: 5 in, 1 out]
        n769 = call "IMAGE ANALYSIS.vi"("Enum"=POST_ANALYSIS_ENUM."OPEN FILE", "error in"=w961, "File Path"=w953) -> ("error out"=w960:errorcluster)  [unwired: 7 in, 1 out]
        n770 = call <vilib>:"Clear Errors.vi"("error in (no error)"=w960) -> ("error out"=w959:errorcluster)  [unwired: 5 in, 1 out]
        n771 = call "IMAGE ANALYSIS.vi"("Enum"=POST_ANALYSIS_ENUM."SHOW UI", "error in"=w959) -> ("error out"=w957:errorcluster)  [unwired: 8 in, 1 out]
        n772 = local write "Zoom Factore"(100.0 ("Zoom Factore")) -> ()
      }
    }
    n773 = case shown="True" w648 {
      selector: w648 -> [_ w936]
      tunnel: w640 -> [w933 w941]
      tunnel: [w933 w935] -> _
      frame False {
      }
      frame True {
        n774 = Not(x=w936) -> (.not. x?=w934:bool)
        n775 = local read "Zoom Factore"() -> (w939:dbl)
        n776 = local write "OUT"(w934) -> ()
        n777 = call "IMAGE ANALYSIS.vi"("Enum"=POST_ANALYSIS_ENUM."ZOOM OUT", "error in"=w941) -> ("error out"=w935:errorcluster)  [unwired: 8 in, 1 out]
        n778 = Divide(x=w939, y=1.2) -> (x/y=w937:dbl)
        n779 = local write "Zoom Factore"(w937) -> ()
      }
    }
    n780 = case shown="True" w649 {
      selector: w649 -> [_ w945]
      tunnel: w640 -> [w942 w950]
      tunnel: [w942 w943] -> _
      frame False {
      }
      frame True {
        n781 = Not(x=w945) -> (.not. x?=w944:bool)
        n782 = local read "Zoom Factore"() -> (w948:dbl)
        n783 = local write "In"(w944) -> ()
        n784 = call "IMAGE ANALYSIS.vi"("Enum"=POST_ANALYSIS_ENUM."ZOOM IN", "error in"=w950) -> ("error out"=w943:errorcluster)  [unwired: 8 in, 1 out]
        n785 = Multiply(x=w948, y=1.2) -> (x*y=w946:dbl)
        n786 = local write "Zoom Factore"(w946) -> ()
      }
    }
    n787 = case shown="True" w645 {
      selector: w645 -> [_ w917]
      tunnel: w640 -> [w915 w919]
      tunnel: [w915 w918] -> _
      frame False {
      }
      frame True {
        n788 = Not(x=w917) -> (.not. x?=w916:bool)
        n789 = local write "Clear ROI Tool"(w916) -> ()
        n790 = call "IMAGE ANALYSIS.vi"("Enum"=POST_ANALYSIS_ENUM."CLEAR ROI", "error in"=w919) -> ("error out"=w918:errorcluster)  [unwired: 8 in, 1 out]
      }
    }
    n791 = case shown="True" w647 {
      selector: w647 -> [_ w929]
      tunnel: w640 -> [w927 w932]
      tunnel: [w927 w930] -> _
      frame False {
      }
      frame True {
        n792 = Not(x=w929) -> (.not. x?=w928:bool)
        n793 = local write "line tool"(w928) -> ()
        n794 = call "IMAGE ANALYSIS.vi"("Enum"=POST_ANALYSIS_ENUM."DRAW LINE", "error in"=w932) -> ("error out"=w930:errorcluster)  [unwired: 8 in, 1 out]
      }
    }
    n795 = case shown="True" w646 {
      selector: w646 -> [_ w923]
      tunnel: w640 -> [w921 w925]
      tunnel: [w921 w924] -> _
      frame False {
      }
      frame True {
        n796 = Not(x=w923) -> (.not. x?=w922:bool)
        n797 = local write "Rectangle Tool"(w922) -> ()
        n798 = call "IMAGE ANALYSIS.vi"("Enum"=POST_ANALYSIS_ENUM."DRAW REC", "error in"=w925) -> ("error out"=w924:errorcluster)  [unwired: 8 in, 1 out]
      }
    }
    n799 = local read "SCAR MEASURMENT"() -> (w633:enum32{"Auto Scar", "Manual Scar"})
    n800 = local read "Fit to Screen Tool"() -> (w642:bool)
    n801 = local read "Resize Tool"() -> (w641:bool)
    n802 = case shown="\"Manual Scar\", Default" w633 {
      frame "Auto Scar" {
        n803 = property on="Cap Live Image" class="Bool (strict)"("BoolText.Text"="Report" ("Boolean Text.Text")) -> ()  [unwired: 2 in, 2 out]
      }
      frame "Manual Scar", Default {
        n804 = property on="Cap Live Image" class="Bool (strict)"("BoolText.Text"="Save Image" ("Boolean Text.Text")) -> ()  [unwired: 2 in, 2 out]
      }
    }
    n805 = local read "ROI Color Tool"() -> (w643:bool)
    n806 = local read "Pan Tool"() -> (w644:bool)
    n807 = case shown="True" w644 {
      selector: w644 -> [_ w911]
      tunnel: w640 -> [w909 w913]
      tunnel: [w909 w912] -> _
      frame False {
      }
      frame True {
        n808 = Not(x=w911) -> (.not. x?=w910:bool)
        n809 = call "IMAGE ANALYSIS.vi"("Enum"=POST_ANALYSIS_ENUM."PAN", "error in"=w913) -> ("error out"=w912:errorcluster)  [unwired: 8 in, 1 out]
        n810 = local write "Pan Tool"(w910) -> ()
      }
    }
    n811 = case shown="True" w641 {
      selector: w641 -> [_ w895]
      tunnel: w640 -> [w890 w892]
      tunnel: [w890 w891] -> _
      frame False {
      }
      frame True {
        n812 = Not(x=w895) -> (.not. x?=w894:bool)
        n813 = local write "Resize Tool"(w894) -> ()
        n814 = call "IMAGE ANALYSIS.vi"("Enum"=POST_ANALYSIS_ENUM."RESIZE MODE", "error in"=w892) -> ("error out"=w891:errorcluster)  [unwired: 8 in, 1 out]
      }
    }
    n815 = case shown="True" w642 {
      selector: w642 -> [_ w900]
      tunnel: [w896 w901] -> _
      tunnel: w640 -> [w896 w899]
      frame False {
      }
      frame True {
        n816 = Not(x=w900) -> (.not. x?=w898:bool)
        n817 = local write "Zoom Factore"(100.0 ("Zoom Factore")) -> ()
        n818 = local write "Fit to Screen Tool"(w898) -> ()
        n819 = call "IMAGE ANALYSIS.vi"("Enum"=POST_ANALYSIS_ENUM."FIT", "error in"=w899) -> ("error out"=w901:errorcluster)  [unwired: 8 in, 1 out]
      }
    }
    n820 = case shown="True" w643 {
      selector: w643 -> [_ w906]
      tunnel: [w903 w907] -> _
      tunnel: w640 -> [w903 w904]
      frame False {
      }
      frame True {
        n821 = Not(x=w906) -> (.not. x?=w905:bool)
        n822 = local write "ROI Color Tool"(w905) -> ()
        n823 = call "IMAGE ANALYSIS.vi"("Enum"=POST_ANALYSIS_ENUM."SET ROI COLOR", "error in"=w904) -> ("error out"=w907:errorcluster)  [unwired: 8 in, 1 out]
      }
    }
    n824 = local read "Quit"() -> (w657:bool)
  }
  n825 = while {
    stop <- w991 stop-if-true
    n826 = local read "Image Path"() -> (w994:path)
    n827 = local read "Print 3"() -> (w997:bool)
    n828 = Equal?(x=w994, y=path "") -> (x = y?=w993:bool)
    n829 = Not(x=w993) -> (.not. x?=w992:bool)
    n830 = property on="Print 3" class="Bool (strict)"("Visible"=w992) -> ()  [unwired: 2 in, 2 out]
    n831 = case shown="True" w997 {
      frame False {
        n832 = local write "Rd"(TRUE ("Boolean 7")) -> ()
      }
      frame True {
        n833 = flat-sequence {
          tunnel: [w1037] -> w1005
          tunnel: [w1024] -> w1003
          tunnel: [w1034] -> w999
          tunnel: w1005 -> [w1046]
          tunnel: [w1046] -> w1004
          tunnel: w1003 -> [w1045]
          tunnel: [w1045] -> w1002
          tunnel: [w1043] -> w1001
          tunnel: [w1042] -> w1000
          tunnel: w999 -> [w1042]
          tunnel: w1004 -> [w1048]
          tunnel: w1002 -> [w1049]
          tunnel: w1001 -> [_]
          tunnel: w1000 -> [w1047]
          frame #0 {
            n834 = case shown="True" "Rd" {
              frame False {
              }
              frame True {
                n835 = while {
                  tunnel: "abcdefABCDEF" ("string 2") -> [w1016]
                  shift-right: [w1014] -> w1008
                  shift-left: "" -> [w1013]
                  i -> [w1023]
                  stop <- w1022 stop-if-true
                  n836 = Random Number (0-1)() -> (number: 0 to 1=w1017:dbl)
                  n837 = Multiply(x=w1017, y=62.0) -> (x*y=w1019:dbl)
                  n838 = Decrement(x="Length 2") -> (x-1=w1012:i16)
                  n839 = To Word Integer(number=w1019) -> (16bit integer=w1020:i16)
                  n840 = String Subset(string=w1016, offset (0)=w1020, length (rest)=1 ("length (rest)")) -> (substring=w1015:string)
                  n841 = Greater Or Equal?(x=w1023, y=w1012) -> (x >= y?=w1022:bool)
                  n842 = Concatenate Strings(w1015, w1013) -> (w1014:string)
                }
                "String 10" <- w1008
                n843 = local write "Rd"(FALSE ("Boolean 7")) -> ()
              }
            }
          }
          frame #1 {
            w1035 = "_resized.jpg" ("command line")
            (unwired) ".jpg -resize 320x240 " ("string")
            (unwired) "Choose an Image File" ("prompt")
            # "-resize 1798x425"
            n844 = local read "Image Path"() -> (w1029:path)
            n845 = Strip Path(path=w1029) -> (stripped path=w1024:path, name=w1025:string)
            n846 = Match Pattern(string=w1025, regular expression=".jpg") -> (before substring=→"before substring 2":string, after substring=→"after substring":string)  [unwired: 1 in, 2 out]
            n847 = Match Pattern(string=w1025, regular expression="\\") -> (before substring=w1031:string)  [unwired: 1 in, 3 out]
            n848 = Match Pattern(string=w1031, regular expression=".jpg") -> (before substring=w1030:string)  [unwired: 1 in, 3 out]
            n849 = Concatenate Strings("cmd /c convert " ("string"), w1030, ".jpg -resize 320x240  " ("command line"), w1030, w1035) -> (w1038:string)
            n850 = call <vilib>:"System Exec.vi"("run minimized? (F)"=TRUE, "wait until completion? (T)"=TRUE, "working directory"=w1024, "command line"=w1038) -> ("error out"=w1037:errorcluster)  [unwired: 4 in, 3 out]
            "error out 2" <- w1037
            n851 = Concatenate Strings(w1030, w1035) -> (w1034:string)
          }
          frame #2 {
            n852 = Wait (ms)(milliseconds to wait=u32 2000 ("millisecond timer value")) -> (millisecond timer value=w1043:u32)
          }
          frame #3 {
            n853 = case shown="No Error" w1048 {
              tunnel: w1049 -> [w1052 _]
              tunnel: w1047 -> [w1050 _]
              frame No Error {
                (unwired) ".jpg" ("string")
                n854 = Path To String(path=w1052) -> (string=w1056:string)
                n855 = Concatenate Strings(w1056, "\\" ("string"), w1050) -> (w1055:string)
                n856 = String To Path(string=w1055) -> (path=w1054:path)
                n857 = call <vilib>:"Read JPEG File.vi"("path to JPEG file"=w1054) -> ("image data"=w1058:T15)  [unwired: 8 in, 2 out]
                "image data" <- w1058
                n858 = local write "Print 3"(FALSE ("Print 2")) -> ()
                n859 = call <vilib>:"Draw Flattened Pixmap.vi"("image data"=w1058) -> ("new picture"=→"new picture":picture)  [unwired: 8 in]
              }
              frame Error {
              }
            }
          }
        }
      }
    }
    n860 = Wait (ms)(milliseconds to wait=u32 20 ("millisecond timer value")) -> ()  [unwired: 1 out]
    n861 = local read "Quit"() -> (w991:bool)
  }
  n862 = while {
    tunnel: w33 -> [_]
    tunnel: w17 -> [_]
    stop <- w1089 stop-if-true
    # "New Adv Logics"
    n863 = local read "Main Tab"() -> (w1069:T2)
    n864 = local read "Main Tab"() -> (w1087:T2)
    n865 = local read "Sign In"() -> (w1086:bool)
    n866 = case shown="\"Adv Scar\"" w1069 {
      frame "HOME", Default {
        n867 = local read "LIVE FEED MIN TEMP"() -> (w1222:bool)
        n868 = local write "LIVE FEED MAX TEMP"(TRUE ("LIVE FEED MAX TEMP")) -> ()
        n869 = local read "CAMERA ROI MIN TEMP"() -> (w1220:bool)
        n870 = case shown="True" w1222 {
          selector: w1222 -> [_ w1229]
          frame False {
          }
          frame True {
            n871 = Not(x=w1229) -> (.not. x?=w1228:bool)
            n872 = local write "LIVE FEED MIN TEMP"(w1228) -> ()
            n873 = call "CAMERA LIVE FEED FGV.vi"("Enum - Menu"=CAMERA_LIVE_FEED_ENUM."CAMERA MINIMIZE") -> ()  [unwired: 9 in, 2 out]
          }
        }
        n874 = case shown="True" w1220 {
          selector: w1220 -> [_ w1226]
          frame False {
          }
          frame True {
            n875 = Not(x=w1226) -> (.not. x?=w1225:bool)
            n876 = local write "CAMERA ROI MIN TEMP"(w1225) -> ()
            n877 = call "IMAGE ANALYSIS.vi"("Enum"=POST_ANALYSIS_ENUM."MINIMIZE UI") -> ()  [unwired: 9 in, 2 out]
          }
        }
        n878 = local write "CAMERA ROI MAX TEMP"(TRUE ("CAMERA ROI MAX TEMP")) -> ()
      }
      frame "Test Setup" {
        n879 = local read "LIVE FEED MIN TEMP"() -> (w1232:bool)
        n880 = local read "CAMERA ROI MIN TEMP"() -> (w1230:bool)
        n881 = local write "LIVE FEED MAX TEMP"(TRUE ("LIVE FEED MAX TEMP")) -> ()
        n882 = case shown="True" w1232 {
          selector: w1232 -> [_ w1239]
          frame False {
          }
          frame True {
            n883 = Not(x=w1239) -> (.not. x?=w1238:bool)
            n884 = local write "LIVE FEED MIN TEMP"(w1238) -> ()
            n885 = call "CAMERA LIVE FEED FGV.vi"("Enum - Menu"=CAMERA_LIVE_FEED_ENUM."CAMERA MINIMIZE") -> ()  [unwired: 9 in, 2 out]
          }
        }
        n886 = case shown="True" w1230 {
          selector: w1230 -> [_ w1236]
          frame False {
          }
          frame True {
            n887 = Not(x=w1236) -> (.not. x?=w1235:bool)
            n888 = local write "CAMERA ROI MIN TEMP"(w1235) -> ()
            n889 = call "IMAGE ANALYSIS.vi"("Enum"=POST_ANALYSIS_ENUM."MINIMIZE UI") -> ()  [unwired: 9 in, 2 out]
          }
        }
        n890 = local write "CAMERA ROI MAX TEMP"(TRUE ("CAMERA ROI MAX TEMP")) -> ()
      }
      frame "Acquire" {
        n891 = local read "LIVE FEED MIN TEMP"() -> (w1242:bool)
        n892 = local write "LIVE FEED MAX TEMP"(TRUE ("LIVE FEED MAX TEMP")) -> ()
        n893 = local read "CAMERA ROI MIN TEMP"() -> (w1240:bool)
        n894 = case shown="True" w1242 {
          selector: w1242 -> [_ w1249]
          frame False {
          }
          frame True {
            n895 = Not(x=w1249) -> (.not. x?=w1248:bool)
            n896 = local write "LIVE FEED MIN TEMP"(w1248) -> ()
            n897 = call "CAMERA LIVE FEED FGV.vi"("Enum - Menu"=CAMERA_LIVE_FEED_ENUM."CAMERA MINIMIZE") -> ()  [unwired: 9 in, 2 out]
          }
        }
        n898 = case shown="True" w1240 {
          selector: w1240 -> [_ w1246]
          frame False {
          }
          frame True {
            n899 = Not(x=w1246) -> (.not. x?=w1245:bool)
            n900 = local write "CAMERA ROI MIN TEMP"(w1245) -> ()
            n901 = call "IMAGE ANALYSIS.vi"("Enum"=POST_ANALYSIS_ENUM."MINIMIZE UI") -> ()  [unwired: 9 in, 2 out]
          }
        }
        n902 = local write "CAMERA ROI MAX TEMP"(TRUE ("CAMERA ROI MAX TEMP")) -> ()
      }
      frame "Adv Scar" {
        n903 = local read "CAMERA ROI MIN TEMP"() -> (w1250:bool)
        n904 = case shown="True" "LIVE FEED MAX TEMP" {
          selector: "LIVE FEED MAX TEMP" -> [_ w1271]
          frame False {
          }
          frame True {
            n905 = Not(x=w1271) -> (.not. x?=w1270:bool)
            n906 = local write "LIVE FEED MAX TEMP"(w1270) -> ()
            n907 = call "CAMERA LIVE FEED FGV.vi"("Enum - Menu"=CAMERA_LIVE_FEED_ENUM."CAMERA RESTORE") -> ("error out"=w1261:errorcluster)  [unwired: 9 in, 1 out]
            n908 = Type Cast(type=30, x=0) -> (*(type *) &x=w1265:i32)
            n909 = Add(x=w1265, y=48) -> (x+y=w1266:i32)
            n910 = call "CAMERA LIVE FEED FGV.vi"("Enum - Menu"=CAMERA_LIVE_FEED_ENUM."CAMERA MODE SET", "error in (no error)"=w1261, "CAMERA MODE"=w1266) -> ("error out"=w1258:errorcluster)  [unwired: 7 in, 1 out]
            n911 = call "CAMERA LIVE FEED FGV.vi"("Enum - Menu"=CAMERA_LIVE_FEED_ENUM."CAMERA GRAY", "error in (no error)"=w1258) -> ("error out"=w1257:errorcluster)  [unwired: 8 in, 1 out]
            n912 = call "LIST FILE NAMES.vi"("error in (no error)"=w1257) -> ("error out"=w1267:errorcluster, "filenames"=w1268:string[])  [unwired: 9 in]
            n913 = property on="FILE 3" class="CmbBox"(error in=w1267, "Strings[]"=w1268) -> ()  [unwired: 1 in, 2 out]
          }
        }
        n914 = case shown="True" w1250 {
          selector: w1250 -> [_ w1256]
          frame False {
          }
          frame True {
            n915 = Not(x=w1256) -> (.not. x?=w1255:bool)
            n916 = local write "CAMERA ROI MIN TEMP"(w1255) -> ()
            n917 = call "IMAGE ANALYSIS.vi"("Enum"=POST_ANALYSIS_ENUM."MINIMIZE UI") -> ()  [unwired: 9 in, 2 out]
          }
        }
        n918 = local write "CAMERA ROI MAX TEMP"(TRUE ("CAMERA ROI MAX TEMP")) -> ()
        "LIVE FEED MIN TEMP" <- TRUE ("LIVE FEED MIN TEMP")
      }
      frame "Adv Scar Report" {
        n919 = local read "CAMERA ROI MAX TEMP"() -> (w1272:bool)
        n920 = local read "LIVE FEED MIN TEMP"() -> (w1274:bool)
        n921 = local write "LIVE FEED MAX TEMP"(TRUE ("LIVE FEED MAX TEMP")) -> ()
        n922 = case shown="True" w1274 {
          selector: w1274 -> [_ w1283]
          frame False {
          }
          frame True {
            n923 = Not(x=w1283) -> (.not. x?=w1282:bool)
            n924 = local write "LIVE FEED MIN TEMP"(w1282) -> ()
            n925 = call "CAMERA LIVE FEED FGV.vi"("Enum - Menu"=CAMERA_LIVE_FEED_ENUM."CAMERA MINIMIZE") -> ()  [unwired: 9 in, 2 out]
          }
        }
        n926 = case shown="True" w1272 {
          selector: w1272 -> [_ w1280]
          frame False {
          }
          frame True {
            n927 = Not(x=w1280) -> (.not. x?=w1278:bool)
            n928 = local write "CAMERA ROI MAX TEMP"(w1278) -> ()
            n929 = call "IMAGE ANALYSIS.vi"("Enum"=POST_ANALYSIS_ENUM."SHOW UI") -> ("error out"=w1277:errorcluster)  [unwired: 9 in, 1 out]
            n930 = call "LIST FILE NAMES.vi"("error in (no error)"=w1277) -> ("filenames"=w1276:string[])  [unwired: 9 in, 1 out]
            n931 = property on="Test File List :" class="CmbBox"("Strings[]"=w1276) -> ()  [unwired: 2 in, 2 out]
          }
        }
        n932 = local write "CAMERA ROI MIN TEMP"(TRUE ("CAMERA ROI MIN TEMP")) -> ()
      }
      frame "Compare Files" {
        n933 = local read "LIVE FEED MIN TEMP"() -> (w1286:bool)
        n934 = local write "LIVE FEED MAX TEMP"(TRUE ("LIVE FEED MAX TEMP")) -> ()
        n935 = local read "CAMERA ROI MIN TEMP"() -> (w1284:bool)
        n936 = case shown="True" w1286 {
          selector: w1286 -> [_ w1293]
          frame False {
          }
          frame True {
            n937 = Not(x=w1293) -> (.not. x?=w1292:bool)
